vi "Path to URL inner.vi"(0 "path":path, 1 "App.TargetOS":T1(ring), 2 "Application:Directory Path":path) -> (3 "url":string)   [LabVIEW 2020]
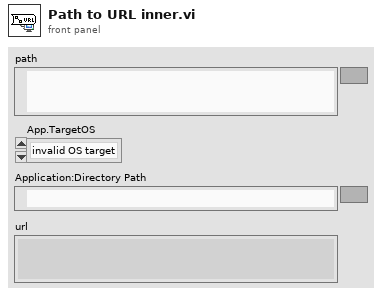
[diagram p1: front panel]
types:
  T1 = enum32{"invalid OS target", "Mac OS", "Windows 3.1", "Windows 95/NT", "Solaris 1", "Solaris 2", "HP-UX", "PowerMAX", "Linux", "Irix", "Rhapsody", "BeOS", "AIX", "OSF1", "VxWorks", "PharLap", "Carbon", "RTX", "Windows x64", "Linux x64", "Mac OS X x64"}
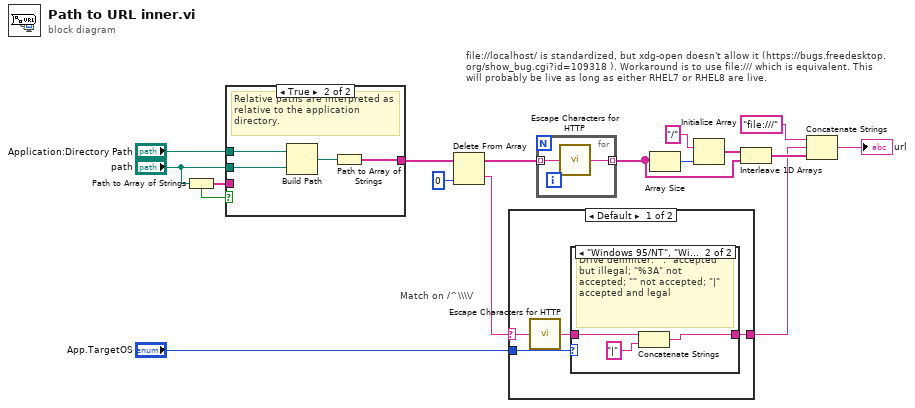
[diagram p0: block diagram]
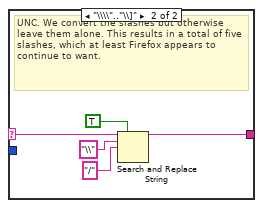
[diagram p3: hidden frame]
diagram:
  # "Match on /^\\\\\\\\/"
  # "file://localhost/ is standardized, but xdg-open doesn't allow it (https://bugs.freedesktop.org/show_bug.cgi?id=109318 ). Workaround is to use file:/// which is equivalent. This will probably be live as long as either RHEL7 or RHEL8 are live."
  n1 = Path to Array of Strings(0:"path") -> (1:w5:bool, 2:w6:string[])
  n2 = case shown="True" w5 {
    tunnel: [w18 w21] -> w7
    tunnel: w6 -> [w18 _]
    tunnel: "path" -> [_ w20]
    tunnel: "Application:Directory Path" -> [_ w19]
    frame False {
    }
    frame True {
      # "Relative paths are interpreted as\nrelative to the application directory."
      n3 = Build Path(base path=w19, name or relative path=w20) -> (appended path=w22:path)
      n4 = Path to Array of Strings(0:w22) -> (2:w21:string[])  [unwired: 1 out]
    }
  }
  n5 = Delete From Array(array=w7, index=0) -> (deleted portion=w10:string, array with subset deleted=w16:string[])  [unwired: 1 in]
  n6 = case shown="Default" w10 {
    selector: w10 -> [w26 w32]
    tunnel: [w23 w31] -> w8
    tunnel: "App.TargetOS" -> [w24 _]
    frame Default {
      n7 = call "Escape Characters for HTTP.vi"("string"=w26) -> ("url-encoded string"=w25:string)
      n8 = case shown="\"Windows 95/NT\", \"Windows x64\"" w24 {
        tunnel: w25 -> [w27 w30]
        tunnel: [w27 w28] -> w23
        frame Default {
        }
        frame "Windows 95/NT", "Windows x64" {
          # "Drive delimiter: '\":\" accepted but illegal; \"%3A\" not accepted; \"\" not accepted; \"|\" accepted and legal"
          n9 = Concatenate Strings(w30, "|" ("string")) -> (w28:string)
        }
      }
    }
    frame "\\\\".."\\]" {
      # "UNC. We convert the slashes but otherwise leave them alone. This results in a total of five slashes, which at least Firefox appears to continue to want."
      n10 = Search and Replace String(replace all?=TRUE ("replace all? (F)"), input string=w32, search string="\\", replace string="/" ("replace string (\"\")")) -> (result string=w31:string)  [unwired: 4 in, 3 out]
    }
  }
  n11 = for {
    tunnel: w16 -> [w37] mode=indexing
    tunnel: [w36] -> w17 mode=indexing
    n12 = call "Escape Characters for HTTP.vi"("string"=w37) -> ("url-encoded string"=w36:string)
  }
  n13 = Array Size(array=w17) -> (size(s)=w12:i32)
  n14 = Initialize Array("/", w12) -> (w14:string[])
  n15 = Interleave 1D Arrays(w14, w17) -> (w15:string[])
  n16 = Concatenate Strings("file:///", w8, w15) -> (→"url":string)
